vi "ParseVI.vi"(11 "VIPath":path) -> (2 "数组":string[][](array[string]), 3 "VIInfo":cluster{"Name":string, "Terminals":T1[]})   [LabVIEW 2018]
uses:
  Ctr/TerminalInfo.ctl
  Ctr/VIInfo.ctl
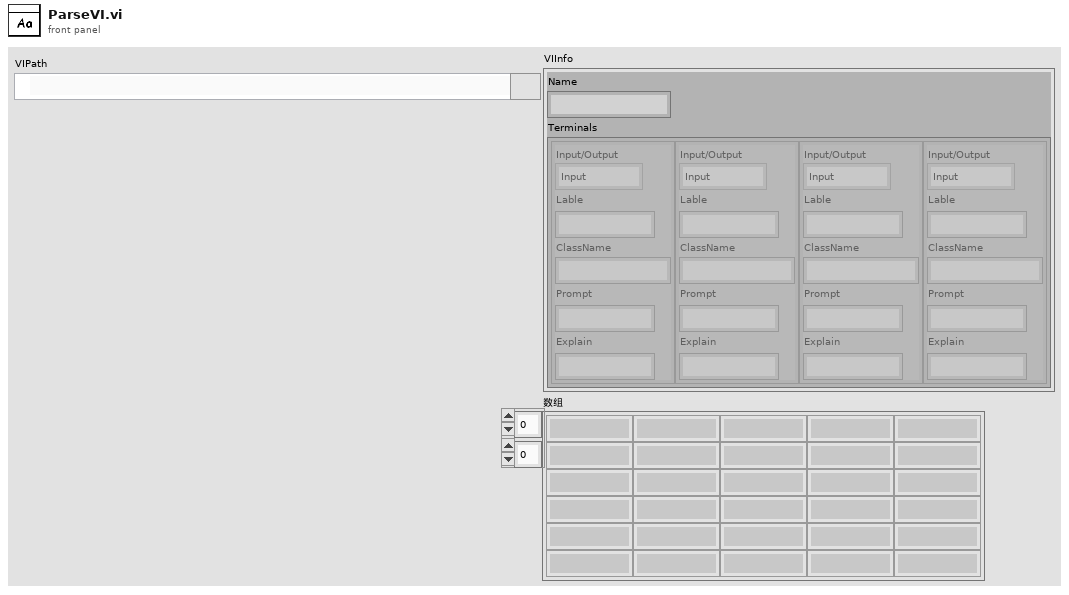
[diagram p1: front panel]
types:
  T1 = typedef "TerminalInfo.ctl" = cluster{"Input/Output":T2, "Lable":string, "ClassName":string, "Prompt":string, "Explain":string}
  T2 = typedef "IsIndicator" = enum16{"Input", "Output"}
  T3 = typedef "VIInfo.ctl" = cluster{"Name":string, "Terminals":T1[]}
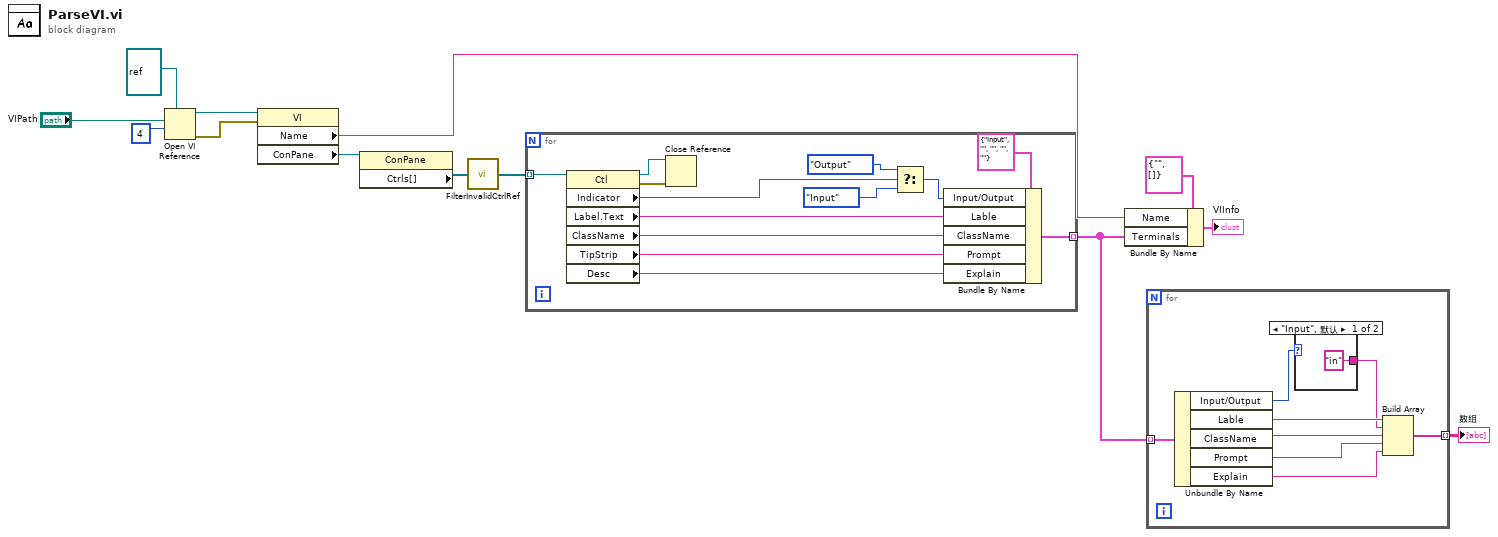
[diagram p0: block diagram]
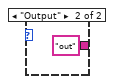
[diagram p2: hidden frame]
diagram:
  n1 = Open VI Reference(type specifier VI Refnum (for type only)=refnum<vi> refnum ("类型说明符VI引用句柄（仅用于类型）"), vi path="VIPath", options=4 ("选项")) -> (vi reference=w8:refnum<vi>, error out=w7:errorcluster)  [unwired: 3 in]
  n2 = property class="VI"(reference=w8, error in=w7) -> ("Name"=w13:string, "ConPane"=w6:refnum<vi>)  [unwired: 2 out]
  n3 = property class="ConPane"(reference=w6) -> ("Ctrls[]"=w4:refnum<vi>[])  [unwired: 1 in, 2 out]
  n4 = call "FilterInvalidCtrlRef.vi"("Ctrls in"=w4) -> ("Ctrl out"=w3:refnum<vi>[])
  n5 = for {
    tunnel: w3 -> [w26] mode=indexing
    tunnel: [w16] -> w2 mode=indexing
    n6 = property class="Ctl"(reference=w26) -> (reference out=w15:refnum<vi>, error out=w14:errorcluster, "Indicator"=w22:bool, "Label.Text"=w23:string, "ClassName"=w24:string, "TipStrip"=w18:string, "Desc"=w17:string)  [unwired: 1 in]
    n7 = Close Reference(reference=w15, error in (no error)=w14) -> ()  [unwired: 1 out]
    n8 = Select(t=IsIndicator."Output" ("Input/Output"), s=w22, f=IsIndicator."Input" ("Input/Output")) -> (s? t:f=w19:T2)
    n9 = Bundle By Name(cluster=T1 {"Input/Output"=enum."Input", "Lable"="", "ClassName"="", "Prompt"="", "Explain"=""} ("NewCluster"), "Input/Output"=w19, "Lable"=w23, "ClassName"=w24, "Prompt"=w18, "Explain"=w17) -> (w16:T1)
  }
  n10 = Bundle By Name(cluster=T3 {"Name"="", "Terminals"=[]} ("输入簇"), "Name"=w13, "Terminals"=w2) -> (→"VIInfo":T3)
  n11 = for {
    tunnel: w2 -> [w34] mode=indexing
    tunnel: [w27] -> w1 mode=indexing
    n12 = Unbundle By Name(w34) -> ("Input/Output"=w29:T2, "Lable"=w33:string, "ClassName"=w30:string, "Prompt"=w31:string, "Explain"=w32:string)
    n13 = case shown="\"Input\", 默认" w29 {
      tunnel: ["in" "out"] -> w28
      frame "Input", Default {
      }
      frame "Output" {
      }
    }
    n14 = Build Array(w33, w28, w30, w31, w32) -> (w27:string[])
  }
  "数组" <- w1
